vi "Trajectory_lerp_Pose.vi"(6 "interpolantFraction":dbl, 9 "endPOSE":T1={"TRANSLATION"={"X"=0.0, "Y"=0.0}, "ROTATION"={"VALUE"=0.0, "COS"=1.0, "SIN"=0.0}} {"ROTATION"."SIN" format="%13.4f"; "ROTATION"."COS" format="%13.4f"; "ROTATION"."VALUE" format="%13.4f"; "TRANSLATION"."Y" format="%14.3f"; "TRANSLATION"."X" format="%14.3f"}, 11 "startPOSE":T1={"TRANSLATION"={"X"=0.0, "Y"=0.0}, "ROTATION"={"VALUE"=0.0, "COS"=1.0, "SIN"=0.0}} {"ROTATION"."SIN" format="%13.4f"; "ROTATION"."COS" format="%13.4f"; "ROTATION"."VALUE" format="%13.4f"; "TRANSLATION"."Y" format="%14.3f"; "TRANSLATION"."X" format="%14.3f"}) -> (3 "outputPOSE":T1={"TRANSLATION"={"X"=0.0, "Y"=0.0}, "ROTATION"={"VALUE"=0.0, "COS"=1.0, "SIN"=0.0}} {"ROTATION"."SIN" format="%13.4f"; "ROTATION"."COS" format="%13.4f"; "ROTATION"."VALUE" format="%13.4f"; "TRANSLATION"."Y" format="%14.3f"; "TRANSLATION"."X" format="%14.3f"})   [LabVIEW 2019, in "Trajectory_Library.lvlib"]
doc: "This is an internal routine. Linearly interpolates between two values.\n\nParameters:\n - startPose - The start Pose.\n - endPose - The end Pose.\n - fraction - The fraction for interpolation.\n\nReturn:\n - outputPose - The interpolated Pose."
uses:
  Trajectory_Library.lvlib
  TypeDef/TRANSLATION2D.ctl
  TypeDef/ROTATION2D.ctl
  TypeDef/POSE2D.ctl
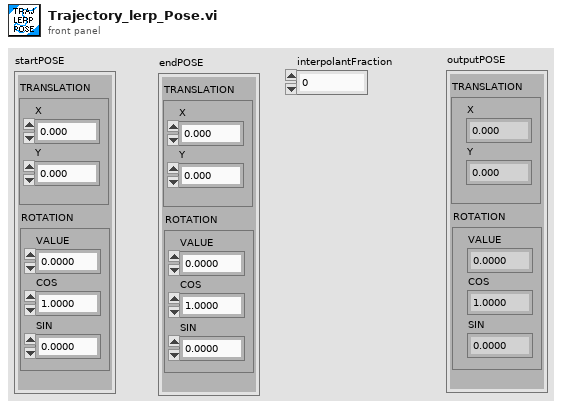
[diagram p1: front panel]
types:
  T1 = typedef "Trajectory_Library.lvlib/POSE2D.ctl" = cluster{"TRANSLATION":T2, "ROTATION":T3}
  T2 = typedef "Trajectory_Library.lvlib/TRANSLATION2D.ctl" = cluster{"X":dbl, "Y":dbl}
  T3 = typedef "Trajectory_Library.lvlib/ROTATION2D.ctl" = cluster{"VALUE":dbl, "COS":dbl, "SIN":dbl}
  T4 = typedef "WPILib_Math.lvlib/TRANSFORM2D.ctl" = cluster{"TRANSLATION":T5, "ROTATION":T6, "xF":bool}
  T5 = typedef "WPILib_Math.lvlib/TRANSLATION2D.ctl" = cluster{"X":dbl, "Y":dbl}
  T6 = typedef "WPILib_Math.lvlib/ROTATION2D.ctl" = cluster{"VALUE":dbl, "COS":dbl, "SIN":dbl}
  T7 = typedef "WPILib_Math.lvlib/POSE2D.ctl" = cluster{"TRANSLATION":T5, "ROTATION":T6}
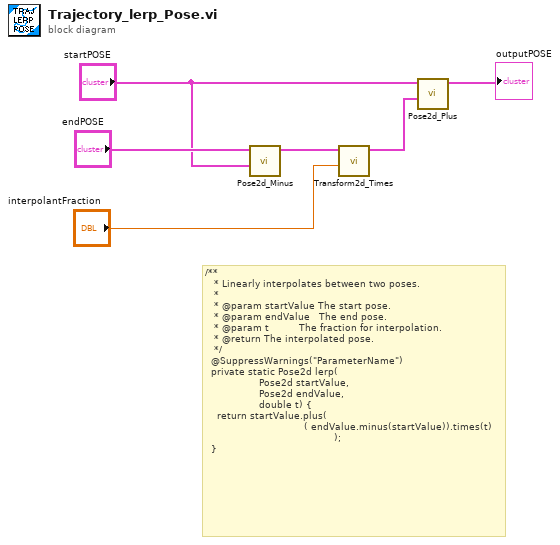
[diagram p0: block diagram]
diagram:
  # "/**\n   * Linearly interpolates between two poses.\n   *\n   * @param startValue The start pose.\n   * @param endValue   The end pose.\n   * @param t          The fraction for interpolation.\n   * @return The interpolated pose.\n   */\n  @SuppressWarnings(\"ParameterName\")\n  private static Pose2d lerp(  \n                  Pose2d startValue, \n                  Pose2d endValue, \n                  double t) {\n    return startValue.plus( \n                                 ( endValue.minus(startValue)).times(t)\n                                           );\n  }"
  n1 = call "Pose2d_Minus.vi"("other POSE"="startPOSE", "in POSE"="endPOSE") -> ("outTRANSFORM"=w5:T4)  [unwired: 9 in]
  n2 = call "Transform2d_Times.vi"("Scalar"="interpolantFraction", "inTRANSFORM"=w5) -> ("TRANSFORM"=w3:T4)  [unwired: 9 in]
  n3 = call "Pose2d_Plus.vi"("other TRANSFORM"=w3, "in POSE"="startPOSE") -> ("out POSE"=→"outputPOSE":T7)  [unwired: 9 in]
